vi "Get Caster Motor Velocity Setpoint.vi"(8 "error in (no error)":errorcluster, 11 "wheel in":refnum<class "NI_Robotics_Caster Wheel.lvclass">) -> (0 "error out":errorcluster, 1 "failed?":bool, 2 "ccw motor velocity setpoint":dbl, 3 "wheel out":refnum<class "NI_Robotics_Caster Wheel.lvclass">)   [LabVIEW 2017, in "NI_Robotics_Caster Wheel.lvclass"]
uses:
  <vilib>/robotics/Steering/Caster Wheel/NI_Robotics_Caster Wheel.lvclass
  <vilib>/robotics/Steering/Caster Wheel/NI_Robotics_Caster Wheel.lvclass/NI_Robotics_Caster Wheel.ctl
  <vilib>/robotics/Actuation/Motor Communication/NI_Robotics_Motor Communication.lvclass
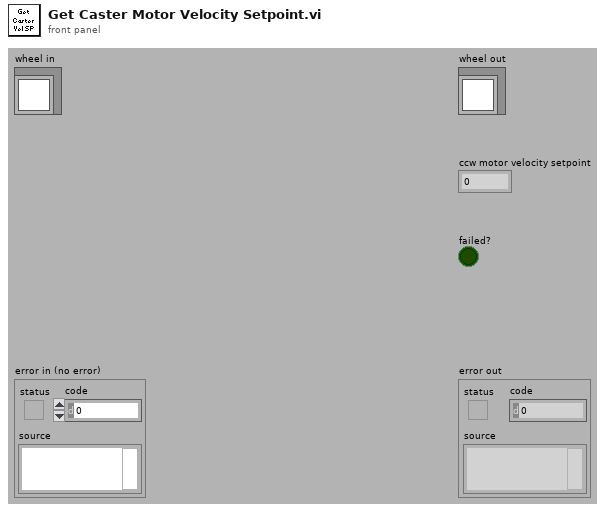
[diagram p1: front panel]
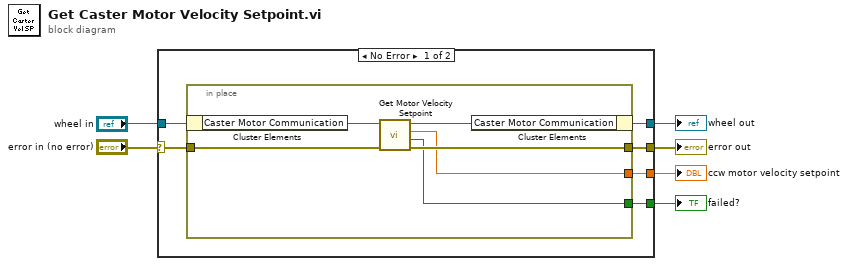
[diagram p0: block diagram]
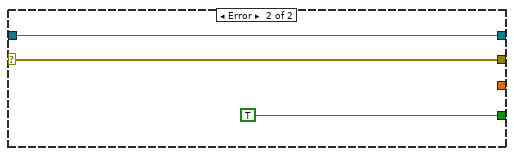
[diagram p2: hidden frame]
diagram:
  n1 = case shown="No Error" "error in (no error)" {
    selector: "error in (no error)" -> [w11 w20]
    tunnel: "wheel in" -> [w12 w21]
    tunnel: [w10 w20] -> w4
    tunnel: [w9 w21] -> w3
    tunnel: [w8 TRUE ("failed?")] -> w2
    tunnel: [w7 _] -> w1
    frame No Error {
      n2 = in-place {
        in-place-border: w11 -> [w16]
        in-place-border: [w15] -> w10
        in-place-border: [w14] -> w8
        in-place-border: [w13] -> w7
        n3 = in-place-cluster #1(w12) -> ("Caster Motor Communication"=w18:refnum<class "NI_Robotics_Motor Communication.lvclass">)
        n4 = call <vilib>:"Get Motor Velocity Setpoint.vi"("error in (no error)"=w16, "motor communication in"=w18) -> ("error out"=w15:errorcluster, "failed?"=w14:bool, "velocity"=w13:dbl, "motor communication out"=w17:refnum<class "NI_Robotics_Motor Communication.lvclass">)  [unwired: 6 in]
        n5 = in-place-cluster #1("Caster Motor Communication"=w17) -> (w9:refnum<class "NI_Robotics_Caster Wheel.lvclass">)
      }
    }
    frame Error {
    }
  }
  "error out" <- w4
  "wheel out" <- w3
  "ccw motor velocity setpoint" <- w1
  "failed?" <- w2
